vi "Format Message String.vi"(9 "ID":string, 10 "Data":string, 11 "Command":string) -> (3 "Message":string)   [LabVIEW 2019, in "RemoteControl.lvclass"]
uses:
  RemoteControl.lvclass
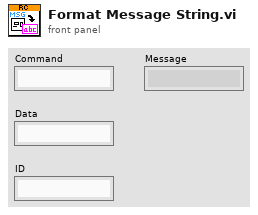
[diagram p1: front panel]
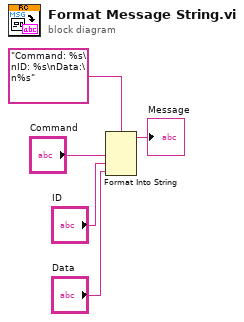
[diagram p0: block diagram]
diagram:
  n1 = Format Into String(format string="Command: %s\nID: %s\nData:\n%s", "Command", "ID", "Data") -> (resulting string=→"Message":string)  [unwired: 2 in, 1 out]
